vi "Get Directions.vi"(11 "Proto in":refnum<class "Directional Keypad.lvclass">) -> (2 "Directional Button Presses":string[](array[string]), 3 "Proto out":refnum<class "Directional Keypad.lvclass">)   [LabVIEW 2020, in "Directional Keypad.lvclass"]
uses:
  Directional Keypad.lvclass
  Directional Keypad.lvclass/Directional Keypad.ctl
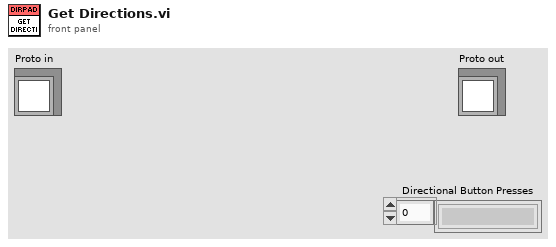
[diagram p1: front panel]
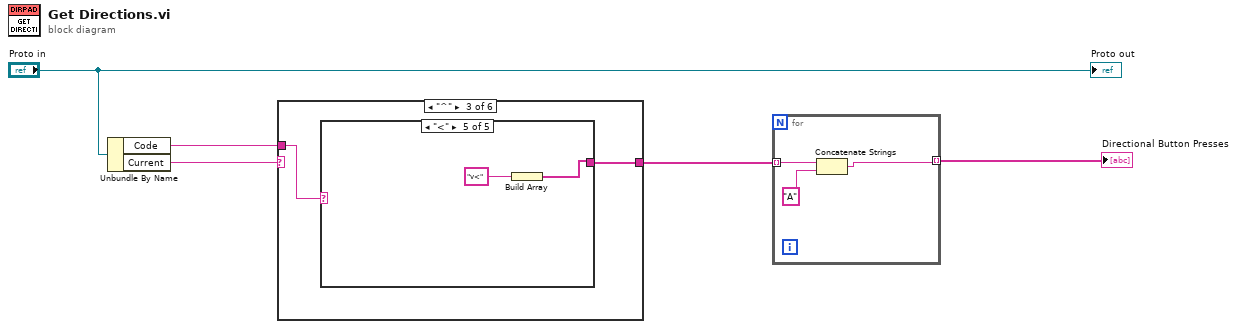
[diagram p0: block diagram]
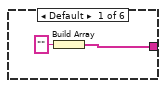
[diagram p2: hidden frame]
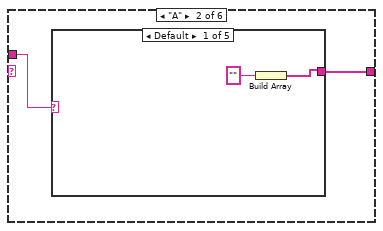
[diagram p3: hidden frame]
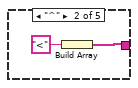
[diagram p4: hidden frame]
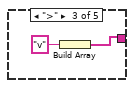
[diagram p5: hidden frame]
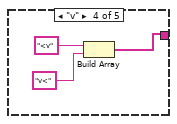
[diagram p6: hidden frame]
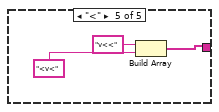
[diagram p7: hidden frame]
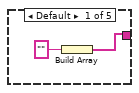
[diagram p8: hidden frame]
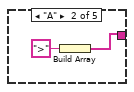
[diagram p9: hidden frame]
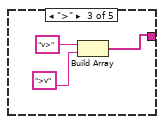
[diagram p10: hidden frame]
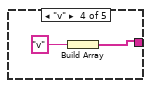
[diagram p11: hidden frame]
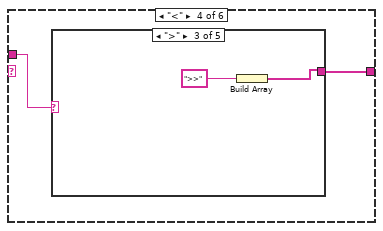
[diagram p12: hidden frame]
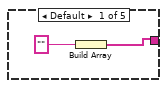
[diagram p13: hidden frame]
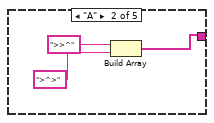
[diagram p14: hidden frame]
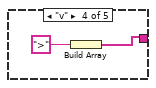
[diagram p15: hidden frame]
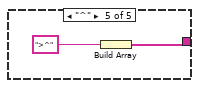
[diagram p16: hidden frame]
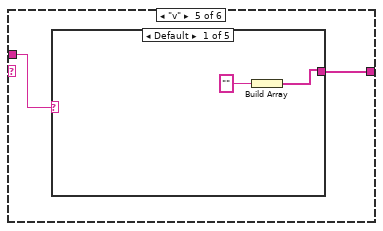
[diagram p17: hidden frame]
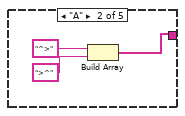
[diagram p18: hidden frame]
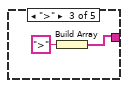
[diagram p19: hidden frame]
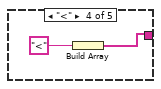
[diagram p20: hidden frame]
diagram:
  n1 = Unbundle By Name("Proto in") -> ("Code"=w2:string, "Current"=w1:string)
  n2 = case shown="\"^\"" w1 {
    tunnel: w2 -> [_ w9 w23 w36 w49 w62]
    tunnel: [w6 w8 w22 w35 w48 w61] -> w3
    frame Default {
      n3 = Build Array("") -> (w6:string[])
    }
    frame "A" {
      n4 = case shown="Default" w9 {
        tunnel: [w10 w12 w14 w17 w20] -> w8
        frame Default {
          n5 = Build Array("") -> (w10:string[])
        }
        frame "^" {
          n6 = Build Array("<") -> (w12:string[])
        }
        frame ">" {
          n7 = Build Array("v") -> (w14:string[])
        }
        frame "v" {
          n8 = Build Array("<v", "v<") -> (w17:string[])
        }
        frame "<" {
          n9 = Build Array("v<<", "<v<") -> (w20:string[])
        }
      }
    }
    frame "^" {
      n10 = case shown="\"<\"" w23 {
        tunnel: [w24 w26 w29 w31 w33] -> w22
        frame Default {
          n11 = Build Array("") -> (w24:string[])
        }
        frame "A" {
          n12 = Build Array(">") -> (w26:string[])
        }
        frame ">" {
          n13 = Build Array("v>", ">v") -> (w29:string[])
        }
        frame "v" {
          n14 = Build Array("v") -> (w31:string[])
        }
        frame "<" {
          n15 = Build Array("v<") -> (w33:string[])
        }
      }
    }
    frame "<" {
      n16 = case shown="\">\"" w36 {
        tunnel: [w37 w40 w42 w44 w46] -> w35
        frame Default {
          n17 = Build Array("") -> (w37:string[])
        }
        frame "A" {
          n18 = Build Array(">>^", ">^>") -> (w40:string[])
        }
        frame ">" {
          n19 = Build Array(">>") -> (w42:string[])
        }
        frame "v" {
          n20 = Build Array(">") -> (w44:string[])
        }
        frame "^" {
          n21 = Build Array(">^") -> (w46:string[])
        }
      }
    }
    frame "v" {
      n22 = case shown="Default" w49 {
        tunnel: [w50 w53 w55 w57 w59] -> w48
        frame Default {
          n23 = Build Array("") -> (w50:string[])
        }
        frame "A" {
          n24 = Build Array("^>", ">^") -> (w53:string[])
        }
        frame ">" {
          n25 = Build Array(">") -> (w55:string[])
        }
        frame "<" {
          n26 = Build Array("<") -> (w57:string[])
        }
        frame "^" {
          n27 = Build Array("^") -> (w59:string[])
        }
      }
    }
    frame ">" {
      n28 = case shown="\"v\"" w62 {
        tunnel: [w63 w65 w67 w69 w72] -> w61
        frame Default {
          n29 = Build Array("") -> (w63:string[])
        }
        frame "A" {
          n30 = Build Array("^") -> (w65:string[])
        }
        frame "v" {
          n31 = Build Array("<") -> (w67:string[])
        }
        frame "<" {
          n32 = Build Array("<<") -> (w69:string[])
        }
        frame "^" {
          n33 = Build Array("<^", "^<") -> (w72:string[])
        }
      }
    }
  }
  n34 = for {
    tunnel: [w76] -> w4 mode=indexing
    tunnel: w3 -> [w75] mode=indexing
    n35 = Concatenate Strings(w75, "A" ("string")) -> (w76:string)
  }
  "Directional Button Presses" <- w4
  "Proto out" <- "Proto in"
